vi "svl_Level Units.vi"(4 "include weighting if dB On FALSE":bool=TRUE, 6 "rms level (T)":bool=TRUE, 7 "channel info":T1={"sensor sensitivity"=1000.0, "engineering units"=1, "dB reference"=1.0, "custom label"="EU", "weighting filter"=0, "pregain"=0.0} {"pregain" format="%.2f"; "weighting filter" items=["Linear", "A-weighting", "B-weighting", "C-weighting", "ITU-R 468-4", "Dolby", "CCITT", "C-message", "Wb", "Wc", "Wd", "We", "Wf", "Wh", "Wj", "Wk", "Wm", "AES17 20 kHz lowpass", "AES17 40 kHz lowpass", "AES17 20 kHz highpass", "AES17 40 kHz highpass"]; "dB reference" format="%^.1e"; "engineering units" items=["custom..."=0, "V"=1, "A"=21, "C"=30, "pC"=31, "s"=32, "-"=29, "Pa"=2, "N"=20, "g"=3, "m/s^2"=4, "m/s"=5, "m"=6, "mm/s"=12, "mm"=13, "micron/s"=14, "micron"=15, "in/s^2"=7, "in/s"=8, "in"=9, "mil/s"=10, "mil"=11, "rad/s^2"=16, "rad/s"=17, "rad"=18, "deg/s^2"=26, "deg/s"=27, "deg"=28, "RPM"=22, "cycle/s^2"=23, "Hz"=24, "cycle"=25, "strain"=19]; "sensor sensitivity" format="%#_5f"}, 8 "error in (no error)":errorcluster, 9 "view mode":enum16{"Power", "Amplitude"}(ring)=enum."Amplitude", 10 "dB On (T)":bool=TRUE) -> (0 "error out":errorcluster, 1 "dB reference [EU]":dbl=nan format="%.2f", 2 "unit label":string)   [LabVIEW 2017]
uses:
  <vilib>/addons/_NISVFA/_Shared subVIs/Controls/svc_Channel Info.ctl
  <vilib>/addons/_NISVFA/_Shared subVIs/Controls/svc_Engineering Units Text Ring.ctl
  <vilib>/addons/_NISVFA/_Shared subVIs/Controls/svc_Weighting Filter Text Ring.ctl
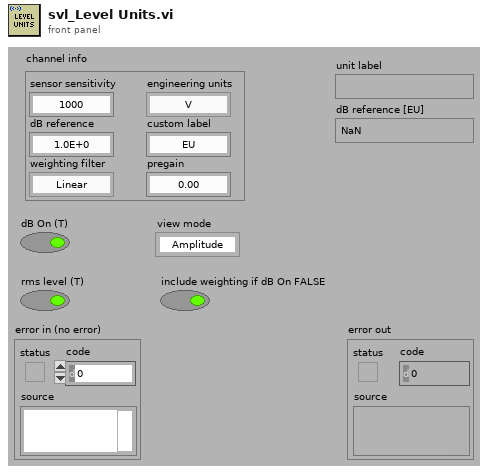
[diagram p1: front panel]
types:
  T1 = typedef "svc_Channel Info.ctl" = cluster{"sensor sensitivity":dbl, "engineering units":T2, "dB reference":dbl, "custom label":string, "weighting filter":T3, "pregain":dbl}
  T2 = typedef "svc_Engineering Units Text Ring.ctl" = u16
  T3 = typedef "svc_Weighting Filter Text Ring.ctl" = u16
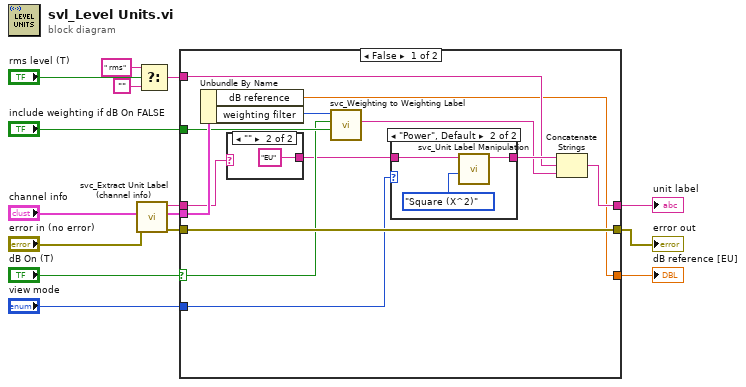
[diagram p0: block diagram]
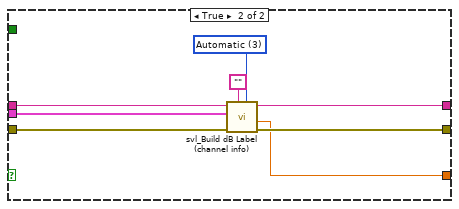
[diagram p4: hidden frame]
diagram:
  n1 = call <vilib>:"svc_Extract Unit Label (channel info).vi"("error in (no error)"="error in (no error)", "channel info"="channel info") -> ("error out"=w9:errorcluster, "channel info"=w11:T1, "unit label"=w10:string)  [unwired: 7 in]
  n2 = Select(t=" rms", s="rms level (T)", f="") -> (s? t:f=w2:string)
  n3 = case shown="False" "dB On (T)" {
    selector: "dB On (T)" -> [w24 _]
    tunnel: "include weighting if dB On FALSE" -> [w25 _]
    tunnel: w11 -> [w27 w42]
    tunnel: w9 -> [w28 w41]
    tunnel: w10 -> [w17 w40]
    tunnel: [w22 w37] -> w7
    tunnel: [w28 w39] -> w6
    tunnel: "view mode" -> [w21 _]
    tunnel: w2 -> [w19 _]
    tunnel: [w18 w38] -> w1
    frame False {
      n4 = Unbundle By Name(w27) -> ("dB reference"=w18:dbl, "weighting filter"=w26:T3)
      n5 = case shown="\"\"" w17 {
        selector: w17 -> [w29 _]
        tunnel: [w29 "EU"] -> w16
        frame Default {
        }
        frame "" {
        }
      }
      n6 = call <vilib>:"svc_Weighting to Weighting Label.vi"("include weighting if dB On False (T)"=w25, "dB On (T)"=w24, "weighting filter"=w26) -> ("weighting string"=w20:string)  [unwired: 7 in, 1 out]
      n7 = case shown="\"Power\", Default" w21 {
        tunnel: [w31 w34] -> w23
        tunnel: w16 -> [w31 w32]
        frame "Amplitude" {
        }
        frame "Power", Default {
          n8 = call <vilib>:"svc_Unit Label Manipulation.vi"("operation"=enum16{"Square (X^2)", "Divide (X/Y)"}."Square (X^2)", "X unit label"=w32) -> ("resulting unit label"=w34:string)  [unwired: 5 in]
        }
      }
      n9 = Concatenate Strings(w23, w19, w20) -> (w22:string)
    }
    frame True {
      w35 = i16 3 items=["Engineering", "Exponential", "Fractional", "Automatic"] ("number format")
      n10 = call <vilib>:"svl_Build dB Label (channel info).vi"("number format"=w35, "peak units"="", "error in (no error)"=w41, "channel info"=w42, "EU label"=w40) -> ("error out"=w39:errorcluster, "dB reference [EU]"=w38:dbl, "dB label"=w37:string)  [unwired: 3 in, 1 out]
    }
  }
  "error out" <- w6
  "unit label" <- w7
  "dB reference [EU]" <- w1
